vi "QueryServer_StartServer.vi"(8 "error in (no error)":errorcluster, 10 "gRPCid":T1, 11 "Server Address":string) -> (0 "error out":errorcluster)   [LabVIEW 2019, in "labview-grpc-query-server.lvlib"]
uses:
  labview-grpc-query-server.lvlib
  labview_query_server.dll
  QueryServer_gRPCid.ctl
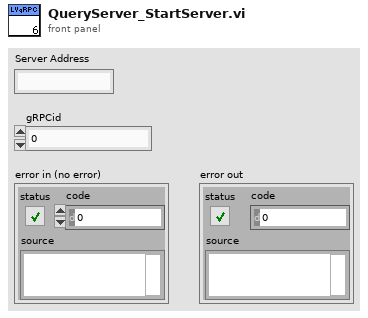
[diagram p1: front panel]
types:
  T1 = typedef "labview-grpc-query-server.lvlib/QueryServer_gRPCid.ctl" = u64
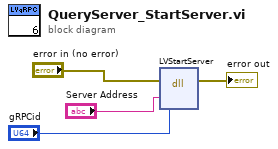
[diagram p0: block diagram]
diagram:
  n1 = dll-call lib="labview_query_server.dll" fn="LVStartServer"(error in="error in (no error)", "serveraddress"="Server Address", "serverid"="gRPCid") -> (error out=→"error out":errorcluster)  [unwired: 5 in, 1 out]
